vi "Magnetic Sweep 1.6.vi"() -> ()   [LabVIEW 2011]
uses:
  <vilib>/Math Plots/3D Math Plots/3D Scatter/3D Scatter XCtrl/3D Scatter.xctl
  <vilib>/Math Plots/3D Math Plots/3D Scatter/3D Scatter Datatype/Public/Plot Helper (Vector).vi
  <vilib>/Math Plots/3D Math Plots/3D Scatter/3D Scatter Datatype/3D Scatter Datatype.lvclass
panel:
  out "3D Scatter (ramp up)":refnum<class "3D Plot Datatype.lvclass">[](xcontrol)
  out "3D Scatter (ramp down)":refnum<class "3D Plot Datatype.lvclass">[](xcontrol)
  out "Heater":bool
  out "Persistent switch ready":bool
  out "error out 6":errorcluster
  in  "Temperature\nlower limite":dbl
  out "Ramping rate command":string
  out "Target field command":string
  out "error out 5":errorcluster
  in  "error out 4":errorcluster
  out "String":string="Persistent switch is not on"
  in  "Set parameter":bool
  out "status":string
  out "PID command":string
  out "setpoint command":string
  out "setpoint":dbl
  in  "stop":bool
  out "error out 3":errorcluster
  out "error out 2":errorcluster
  in  "Contour plot (ramp down)":path
  in  "Raw data (ramp down)":path
  out "Elapsed Time (s)":dbl
  out "Iteration":i32
  in  "error out":errorcluster
  out "Initial Temperature":string
  out "Zero field reached":bool
  out "Target field reached":bool
  in  "Temperature\nupper limite":dbl
  in  "Temperature\nramping step":dbl
  in  "Heater range":i16(ring) items=["High", "Medium", "Low"]
  in  "D gain":dbl
  in  "I gain":dbl
  in  "P gain":dbl
  in  "Contour plot (ramp up)":path
  out "Time elapsed":string
  in  "Timer":bool caption="Reset"
  in  "date format":enum16{"short", "long", "abbreviated"}(ring)
  in  "Save":bool
  in  "Raw data (ramp  up)":path
  out "Temperature vs Time":cluster{dbl[], dbl[]}(graph)
  out "current time":timestamp
  out "Magnetic\nField":cluster{dbl[], dbl[]}(graph)
  out "Current Resistance":string
  out "Current Temperature":string
  out "Current Field":string
  out "Status":string
  in  "Field Sweep":bool
  in  "Magnetic field\nRamp rate":dbl
  in  "Traget Field":dbl
  out "Init Response":string
  in  "error in (no error)":errorcluster
  in  "IP Address":string
  in  "Ramp":bool
  in  "Update":bool
  in  "Ramp to Zero":bool
  in  "P Switch":bool
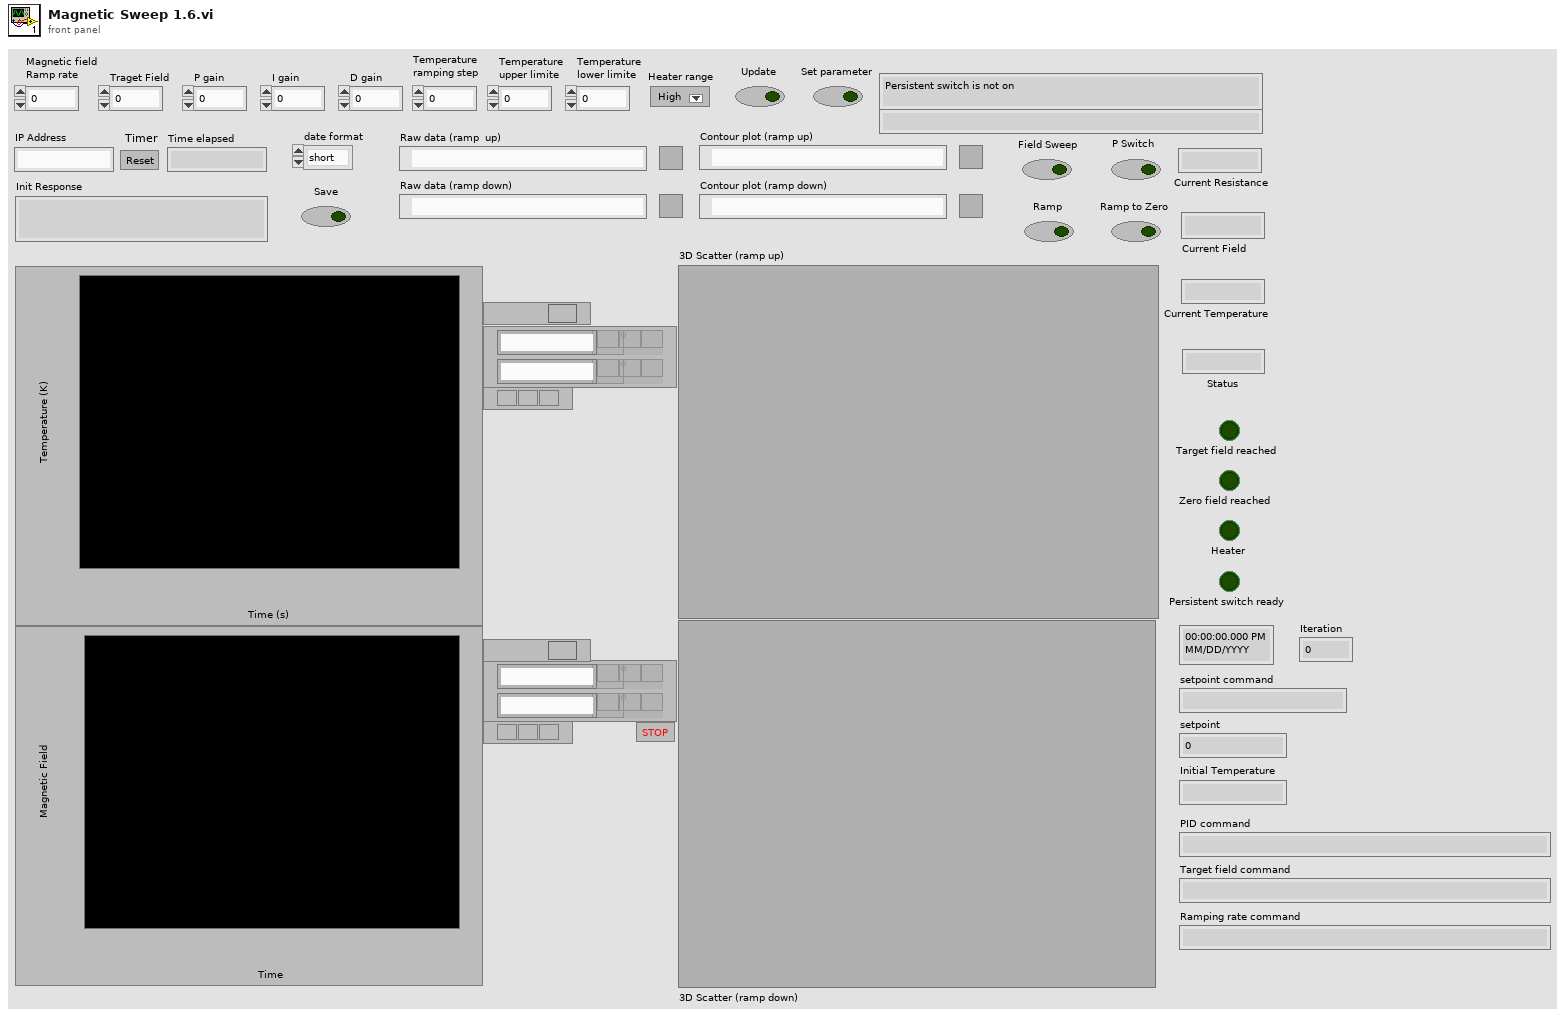
[diagram p1: front panel]
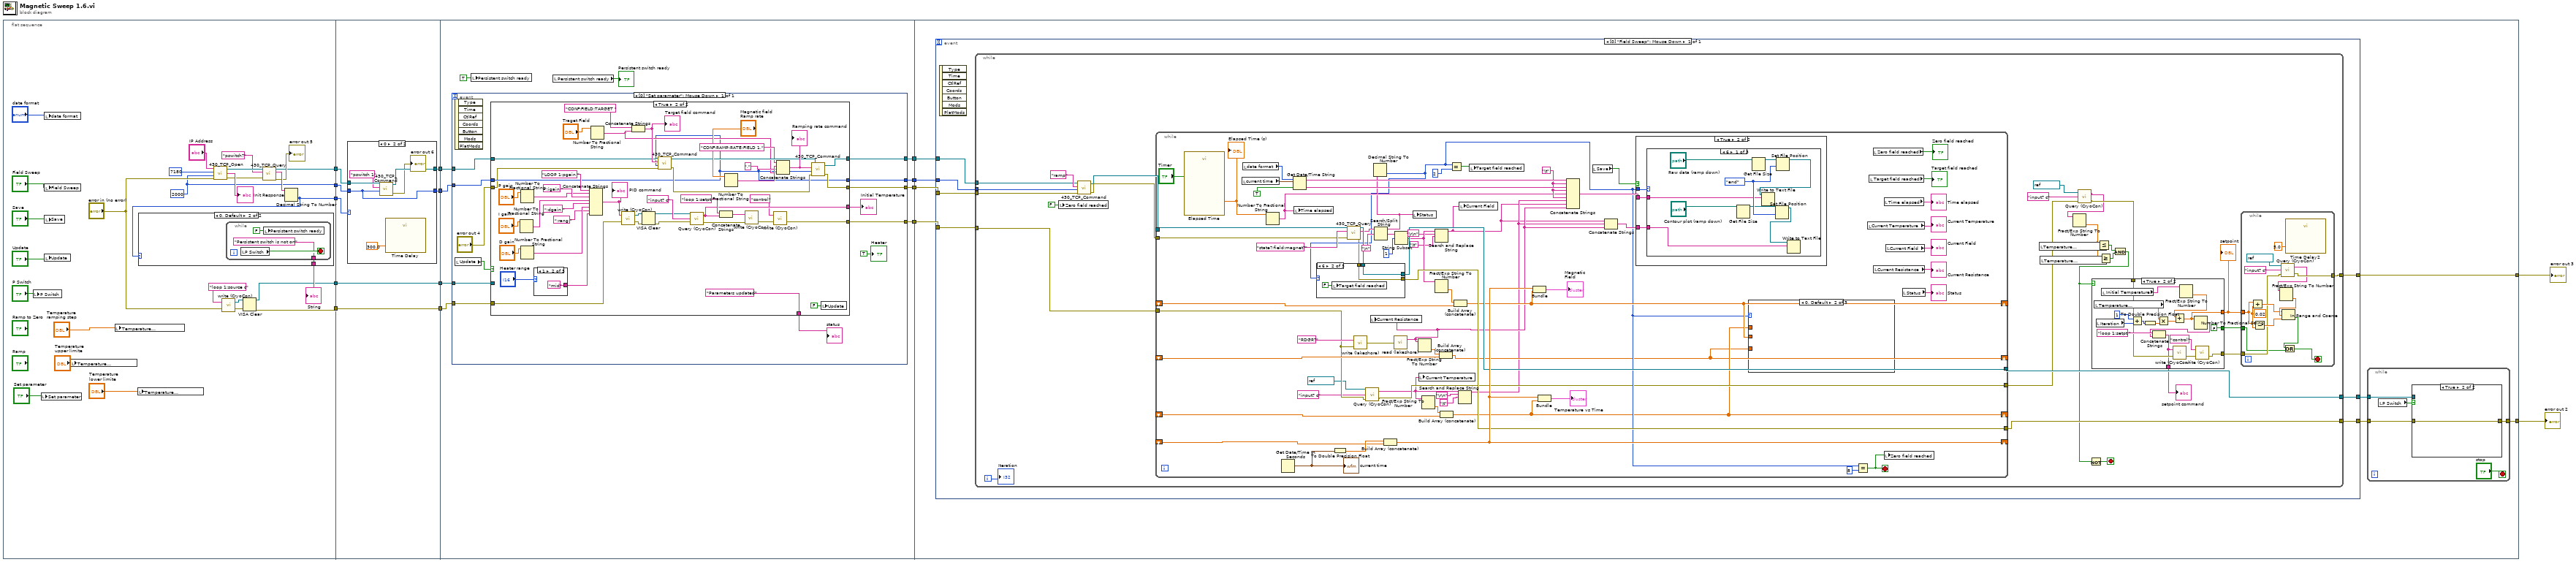
[diagram p0: block diagram]
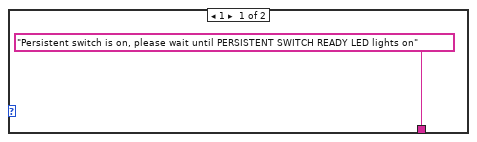
[diagram p2: hidden frame]
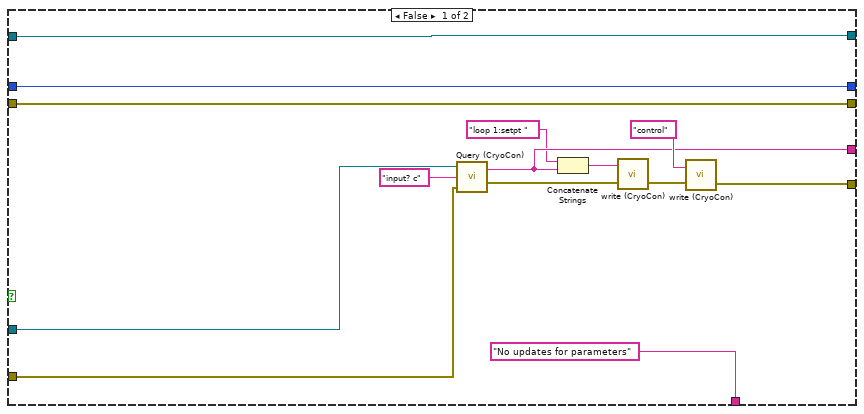
[diagram p4: hidden frame]
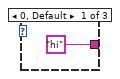
[diagram p5: hidden frame]
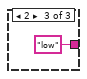
[diagram p6: hidden frame]
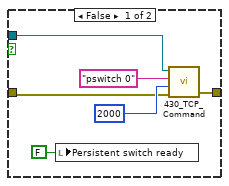
[diagram p7: hidden frame]
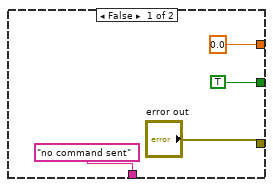
[diagram p8: hidden frame]
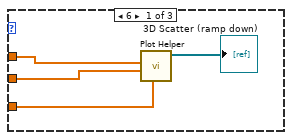
[diagram p9: hidden frame]
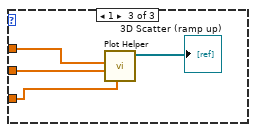
[diagram p10: hidden frame]
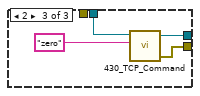
[diagram p12: hidden frame]
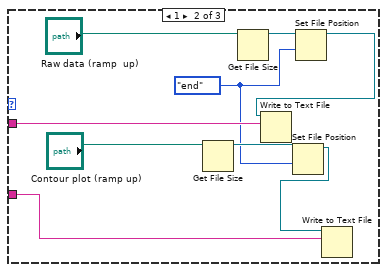
[diagram p14: hidden frame]
diagram:
  n1 = flat-sequence {
    tunnel: [w17] -> w9
    tunnel: [w20] -> w7
    tunnel: [w23] -> w5
    tunnel: [w21] -> w3
    tunnel: [w16] -> w1
    tunnel: w9 -> [w52]
    tunnel: [w50] -> w8
    tunnel: w7 -> [w51]
    tunnel: [w48] -> w6
    tunnel: w5 -> [w54]
    tunnel: [w54] -> w4
    tunnel: w3 -> [w53]
    tunnel: [w53] -> w2
    tunnel: w1 -> [w49]
    tunnel: w8 -> [w72]
    tunnel: w6 -> [w71]
    tunnel: w4 -> [w70]
    tunnel: [w69] -> w15
    tunnel: [w68] -> w12
    tunnel: [w67] -> w11
    tunnel: [w66] -> w10
    tunnel: w2 -> [w65]
    tunnel: w15 -> [w154]
    tunnel: [w153] -> w14
    tunnel: [w151] -> w13
    tunnel: w12 -> [w149]
    tunnel: w11 -> [w148]
    tunnel: w10 -> [w147]
    frame #0 {
      w20 = 2000 ("Timeout")
      n2 = local write "P Switch"("P Switch") -> ()
      n3 = local write "Set parameter"("Set parameter") -> ()
      n4 = local write "date format"("date format") -> ()
      n5 = local write "Field Sweep"("Field Sweep") -> ()
      n6 = local write "Save"("Save") -> ()
      n7 = local write "Update"("Update") -> ()
      n8 = local write "Temperature\nupper limite"("Temperature\nupper limite") -> ()
      n9 = local write "Temperature\nramping step"("Temperature\nramping step") -> ()
      n10 = local write "Temperature\nlower limite"("Temperature\nlower limite") -> ()
      n11 = call "430_TCP_Open.vi"("IP Address"="IP Address", "TCP Port"=7180, "timeout ms (2000)"=w20, "error in (no error)"="error in (no error)") -> ("connection ID"=w30:refnum<k5>, "Init Response"=→"Init Response":string, "error out"=w29:errorcluster)  [unwired: 2 in]
      n12 = call "write (CryoCon).vi"("error in (no error)"="error in (no error)", "write buffer"="loop 1:source c") -> ("error out"=w25:errorcluster, "VISA resource name out"=w24:refnum<visa-resource-name>)
      n13 = VISA Clear(VISA resource name=w24, error in (no error)=w25) -> (VISA resource name out=w21:refnum<visa-resource-name>, error out=w23:errorcluster)
      n14 = call "430_TCP_Query.vi"("error in (no error)"=w29, "Command"="pswitch?", "connection ID"=w30) -> ("error out"=→"error out 5":errorcluster, "Response"=w27:string, "connection ID out"=w17:refnum<k5>)  [unwired: 4 in, 2 out]
      n15 = Decimal String To Number(string=w27) -> (number=w16:i32)  [unwired: 2 in, 1 out]
      n16 = case shown="0, Default" w16 {
        tunnel: ["Persistent switch is on, please wait until PERSISTENT SWITCH READY LED lights on" w44] -> w22
        frame 1 {
        }
        frame 0, Default {
          n17 = while {
            tunnel: ["Persistent switch is not on"] -> w44
            stop <- w47 stop-if-true
            n18 = local read "P Switch"() -> (w47:bool)
            n19 = local write "Persistent switch ready"(FALSE ("Persistent switch ready")) -> ()
          }
        }
      }
      "String" <- w22
    }
    frame #1 {
      n20 = case shown="0" w49 {
        tunnel: w52 -> [w56 w62]
        tunnel: w51 -> [w55 w57]
        tunnel: [w56 w61] -> w50
        tunnel: [w55 w57] -> w48
        frame 1, Default {
        }
        frame 0 {
          n21 = call "430_TCP_Command.vi"("Timeout"=w57, "Command"="pswitch 1", "connection ID"=w62) -> ("error out"=→"error out 6":errorcluster, "connection ID out"=w61:refnum<k5>)  [unwired: 1 in, 1 out]
          n22 = call "Time Delay"("Delay Time (s)"=300.0) -> ()  [unwired: 10 in, 1 out]
        }
      }
    }
    frame #2 {
      n23 = event shown="[0] \"Set parameter\": Mouse Down" {
        selector: _ -> [_]
        dyn-events: _ -> [_]
        timeout: _ -> [_]
        tunnel: w72 -> [w85]
        tunnel: w71 -> [w84]
        tunnel: w70 -> [w83]
        tunnel: [w82] -> w69
        tunnel: [w81] -> w68
        tunnel: [w80] -> w67
        tunnel: [w79] -> w66
        tunnel: w65 -> [w75]
        event "Set parameter": Mouse Down {
          n24 = event-data() -> ()  [unwired: 1 in, 7 out]
          n25 = local read "Update"() -> (w76:bool)
          n26 = case shown="True" w76 {
            tunnel: w85 -> [w97 w141]
            tunnel: w84 -> [w98 w113]
            tunnel: w83 -> [w94 w120]
            tunnel: [w86 w101] -> w82
            tunnel: ["No updates for parameters" ("String") "Parameters updated" ("String")] -> w78
            tunnel: [w93 w115] -> w81
            tunnel: [w97 w114] -> w80
            tunnel: [w98 w113] -> w79
            tunnel: [w89 w105] -> w77
            tunnel: w75 -> [w95 _]
            tunnel: "error out 4" -> [w93 w100]
            frame False {
              n27 = call "Query (CryoCon).vi"("error in (no error)"=w94, "write buffer"="input? c", "VISA resource name 2"=w95) -> ("error out"=w87:errorcluster, "read buffer"=w89:string)
              n28 = Concatenate Strings("loop 1:setpt " ("write buffer"), w89) -> (w92:string)
              n29 = call "write (CryoCon).vi"("error in (no error)"=w87, "write buffer"=w92) -> ("error out"=w91:errorcluster)  [unwired: 1 out]
              n30 = call "write (CryoCon).vi"("error in (no error)"=w91, "write buffer"="control") -> ("error out"=w86:errorcluster)  [unwired: 1 out]
            }
            frame True {
              n31 = Number To Fractional String(number="I gain") -> (F-format string=w124:string)  [unwired: 3 in]
              n32 = Number To Fractional String(number="D gain") -> (F-format string=w122:string)  [unwired: 3 in]
              n33 = Number To Fractional String(number="P gain") -> (F-format string=w125:string)  [unwired: 3 in]
              n34 = case shown="1" "Heater range" {
                tunnel: ["hi" "mid" "low"] -> w117
                frame 0, Default {
                }
                frame 1 {
                }
                frame 2 {
                }
              }
              n35 = Concatenate Strings("LOOP 1:pgain " ("write buffer"), w125, ";igain " ("string"), w124, ";dgain " ("string"), w122, ";rang " ("string"), w117) -> (w121:string)
              "PID command" <- w121
              n36 = Number To Fractional String(number="Traget Field") -> (F-format string=w131:string)  [unwired: 3 in]
              n37 = call "write (CryoCon).vi"("error in (no error)"=w120, "write buffer"=w121) -> ("error out"=w112:errorcluster, "VISA resource name out"=w111:refnum<visa-resource-name>)
              n38 = Concatenate Strings("CONF:FIELD:TARGET ", w131) -> (w142:string)
              "Target field command" <- w142
              n39 = VISA Clear(VISA resource name=w111, error in (no error)=w112) -> (VISA resource name out=w108:refnum<visa-resource-name>, error out=w109:errorcluster)
              n40 = call "430_TCP_Command.vi"("error in (no error)"=w100, "Timeout"=w113, "Command"=w142, "connection ID"=w141) -> ("error out"=w140:errorcluster, "connection ID out"=w136:refnum<k5>)  [unwired: 1 out]
              n41 = call "Query (CryoCon).vi"("error in (no error)"=w109, "write buffer"="input? c", "VISA resource name 2"=w108) -> ("error out"=w107:errorcluster, "read buffer"=w105:string)
              n42 = Concatenate Strings("loop 1:setpt " ("write buffer"), w105) -> (w104:string)
              n43 = Number To Fractional String(number="Magnetic field\nRamp rate") -> (F-format string=w134:string)  [unwired: 3 in]
              n44 = call "write (CryoCon).vi"("error in (no error)"=w107, "write buffer"=w104) -> ("error out"=w103:errorcluster)  [unwired: 1 out]
              n45 = call "write (CryoCon).vi"("error in (no error)"=w103, "write buffer"="control") -> ("error out"=w101:errorcluster)  [unwired: 1 out]
              n46 = Concatenate Strings("CONF:RAMP:RATE:FIELD 1," ("string"), w134, "," ("string"), w131) -> (w137:string)
              "Ramping rate command" <- w137
              n47 = call "430_TCP_Command.vi"("error in (no error)"=w140, "Timeout"=w113, "Command"=w137, "connection ID"=w136) -> ("error out"=w115:errorcluster, "connection ID out"=w114:refnum<k5>)  [unwired: 1 out]
              n48 = local write "Update"(FALSE ("Update")) -> ()
            }
          }
          "Initial Temperature" <- w77
          "status" <- w78
          "Heater" <- TRUE ("Heater")
        }
      }
      n49 = local write "Persistent switch ready"(TRUE ("Persistent switch ready")) -> ()
      n50 = local read "Persistent switch ready"() -> (→"Persistent switch ready":bool)
    }
    frame #3 {
      n51 = event shown="[0] \"Field Sweep\": Mouse Down" {
        selector: _ -> [_]
        dyn-events: _ -> [_]
        timeout: _ -> [_]
        tunnel: w154 -> [w173]
        tunnel: [w172] -> w153
        tunnel: [w171] -> w152
        tunnel: [w170] -> w150
        tunnel: w149 -> [w169]
        tunnel: w148 -> [w168]
        tunnel: w147 -> [w167]
        event "Field Sweep": Mouse Down {
          n52 = event-data() -> ()  [unwired: 1 in, 7 out]
          n53 = while {
            tunnel: w173 -> [w199]
            tunnel: [w191] -> w172
            tunnel: [w190] -> w171
            tunnel: [w189] -> w170
            tunnel: w169 -> [w187]
            tunnel: w168 -> [w186]
            tunnel: w167 -> [w185]
            i -> [w196]
            stop <- w192 stop-if-true
            n54 = local write "Zero field reached"(FALSE ("Zero field reached")) -> ()
            n55 = call "430_TCP_Command.vi"("error in (no error)"=w187, "Timeout"=w185, "Command"="ramp", "connection ID"=w186) -> ("error out"=w201:errorcluster, "connection ID out"=w200:refnum<k5>)  [unwired: 1 out]
            n56 = while {
              shift-right: [w256] -> _
              shift-left: _ -> [w296]
              shift-right: [w243] -> _
              shift-left: _ -> [w301]
              shift-right: [w242] -> _
              shift-left: _ -> [w298]
              shift-right: [w293] -> _
              shift-left: _ -> [w239]
              tunnel: w201 -> [w283]
              tunnel: w200 -> [w282]
              tunnel: w199 -> [w253]
              tunnel: [w252] -> w183
              tunnel: [w264] -> w190
              tunnel: [w263] -> w189
              stop <- w266 stop-if-true
              w287 = "\t"
              n57 = call "Elapsed Time"("Reset"="Timer") -> ("Elapsed Time (s)"=w277:dbl)  [unwired: 11 in, 7 out]
              "Elapsed Time (s)" <- w277
              n58 = local read "current time"() -> (w285:timestamp)
              n59 = local read "date format"() -> (w279:enum16{"short", "long", "abbreviated"})
              n60 = Number To Fractional String(number=w277) -> (F-format string=w280:string)  [unwired: 3 in]
              n61 = Get Date/Time In Seconds() -> (seconds since 1Jan1904=w276:timestamp)
              "current time" <- w276
              n62 = Get Date/Time String(date format (0)=w279, seconds (now)=w285, want seconds? (F)=TRUE) -> (date string=w289:string, time string=w288:string)
              n63 = local write "Time elapsed"(w280) -> ()
              n64 = To Double Precision Float(number=w276) -> (double precision float=w240:dbl)
              n65 = call "430_TCP_Query.vi"("error in (no error)"=w283, "Command"="state?;field:magnet?", "connection ID"=w282) -> ("error out"=w254:errorcluster, "Response"=w262:string, "connection ID out"=w265:refnum<k5>)  [unwired: 4 in, 2 out]
              n66 = call "write (lakeshore).vi"("error in (no error)"=w253, "write buffer"="RDGR?") -> ("error out"=w300:errorcluster)
              n67 = call "Query (CryoCon).vi"("error in (no error)"=w253, "write buffer"="input? c", "VISA resource name 2"=refnum<visa-resource-name> "COM3") -> ("error out"=w252:errorcluster, "read buffer"=w249:string)
              n68 = Search/Split String(string=w262, search string/char (-)="\n") -> (substring before match=w261:string, match + rest of string=w260:string)  [unwired: 1 in, 1 out]
              n69 = Decimal String To Number(string=w261) -> (number=w255:i32)  [unwired: 2 in, 1 out]
              n70 = case shown="6" w255 {
                tunnel: [w311 w313 w318] -> w263
                tunnel: w265 -> [w312 w315 w317]
                tunnel: [w312 w315 w316] -> w264
                tunnel: w254 -> [w311 w313 _]
                frame 0, Default {
                }
                frame 6 {
                  n71 = local write "Target field reached"(FALSE ("Target field reached")) -> ()
                }
                frame 2 {
                  n72 = call "430_TCP_Command.vi"("Command"="zero", "connection ID"=w317) -> ("error out"=w318:errorcluster, "connection ID out"=w316:refnum<k5>)  [unwired: 2 in, 1 out]
                }
              }
              n73 = Build Array (concatenate)(w240, w239) -> (w293:dbl[])
              n74 = call "read (lakeshore).vi"("error in (no error)"=w300) -> ("read buffer"=w241:string)  [unwired: 1 out]
              n75 = local write "Current Resistance"(w241) -> ()
              n76 = String Subset(string=w260, offset (0)=1) -> (substring=w246:string)  [unwired: 1 in]
              n77 = local write "Status"(w261) -> ()
              n78 = Fract/Exp String To Number(string=w241) -> (number=w294:dbl)  [unwired: 3 in, 1 out]
              n79 = local write "Current Temperature"(w249) -> ()
              n80 = Fract/Exp String To Number(string=w249) -> (number=w295:dbl)  [unwired: 3 in, 1 out]
              n81 = Search and Replace String(input string=w246, search string="\r\n", replace string="\t") -> (result string=w237:string)  [unwired: 5 in, 3 out]
              n82 = Fract/Exp String To Number(string=w246) -> (number=w297:dbl)  [unwired: 3 in, 1 out]
              n83 = Build Array (concatenate)(w294, w298) -> (w242:dbl[])
              n84 = Build Array (concatenate)(w295, w301) -> (w243:dbl[])
              n85 = Equal?(x=w255, y=2) -> (x = y?=w281:bool)
              n86 = Build Array (concatenate)(w297, w296) -> (w256:dbl[])
              n87 = Search and Replace String(input string=w249, search string="\r\n", replace string="\t") -> (result string=w238:string)  [unwired: 5 in, 3 out]
              n88 = local write "Current Field"(w237) -> ()
              n89 = local write "Target field reached"(w281) -> ()
              n90 = Bundle(w293, w256) -> (→"Magnetic\nField":cluster{dbl[], dbl[]})  [unwired: 1 in]
              n91 = Bundle(w293, w243) -> (→"Temperature vs Time":cluster{dbl[], dbl[]})  [unwired: 1 in]
              n92 = Concatenate Strings(w289, w287, w288, w287, w280, w287, w238, w237, w241) -> (w292:string)
              n93 = local read "Save"() -> (w275:bool)
              n94 = Concatenate Strings(w237, w238, w241) -> (w286:string)
              n95 = case shown="True" w275 {
                tunnel: w292 -> [_ w322]
                tunnel: w286 -> [_ w321]
                tunnel: w255 -> [_ w320]
                frame False {
                }
                frame True {
                  n96 = case shown="6" w320 {
                    tunnel: w322 -> [w324 w340 _]
                    tunnel: w321 -> [w323 w334 _]
                    frame 6 {
                      w330 = enum16{"start", "end", "current"}."end" ("from (0:start)")
                      n97 = Get File Size(file="Contour plot (ramp down)") -> (refnum out=w329:refnum<file>)  [unwired: 1 in, 2 out]
                      n98 = Get File Size(file="Raw data (ramp down)") -> (refnum out=w326:refnum<file>)  [unwired: 1 in, 2 out]
                      n99 = Set File Position(refnum=w329, from (0:start)=w330) -> (refnum out=w331:refnum<file>)  [unwired: 2 in, 1 out]
                      n100 = Set File Position(refnum=w326, from (0:start)=w330) -> (refnum out=w327:refnum<file>)  [unwired: 2 in, 1 out]
                      n101 = Write to Text File(file (use dialog)=w327, text=w324) -> ()  [unwired: 2 in, 3 out]
                      n102 = Write to Text File(file (use dialog)=w331, text=w323) -> ()  [unwired: 2 in, 3 out]
                    }
                    frame 1 {
                      w333 = enum16{"start", "end", "current"}."end" ("from (0:start)")
                      n103 = Get File Size(file="Contour plot (ramp up)") -> (refnum out=w335:refnum<file>)  [unwired: 1 in, 2 out]
                      n104 = Get File Size(file="Raw data (ramp  up)") -> (refnum out=w338:refnum<file>)  [unwired: 1 in, 2 out]
                      n105 = Set File Position(refnum=w335, from (0:start)=w333) -> (refnum out=w332:refnum<file>)  [unwired: 2 in, 1 out]
                      n106 = Set File Position(refnum=w338, from (0:start)=w333) -> (refnum out=w337:refnum<file>)  [unwired: 2 in, 1 out]
                      n107 = Write to Text File(file (use dialog)=w337, text=w340) -> ()  [unwired: 2 in, 3 out]
                      n108 = Write to Text File(file (use dialog)=w332, text=w334) -> ()  [unwired: 2 in, 3 out]
                    }
                    frame Default {
                    }
                  }
                }
              }
              n109 = case shown="0, Default" w255 {
                tunnel: w243 -> [w304 _ w307]
                tunnel: w256 -> [w303 _ w308]
                tunnel: w242 -> [w305 _ w309]
                frame 6 {
                  n110 = call-poly <vilib>:"Plot Helper.vi"("z vector"=w305, "y vector"=w303, "x vector"=w304) -> ("3D Plot lvclass Array out"=→"3D Scatter (ramp down)":refnum<class "3D Plot Datatype.lvclass">[])  [unwired: 3 in, 5 out]
                }
                frame 0, Default {
                }
                frame 1 {
                  n111 = call-poly <vilib>:"Plot Helper.vi"("z vector"=w309, "y vector"=w308, "x vector"=w307) -> ("3D Plot lvclass Array out"=→"3D Scatter (ramp up)":refnum<class "3D Plot Datatype.lvclass">[])  [unwired: 3 in, 5 out]
                }
              }
              n112 = Equal?(x=w255, y=8) -> (x = y?=w266:bool)
              n113 = local read "Current Temperature"() -> (→"Current Temperature":string)
              n114 = local read "Target field reached"() -> (→"Target field reached":bool)
              n115 = local read "Zero field reached"() -> (→"Zero field reached":bool)
              n116 = local read "Current Resistance"() -> (→"Current Resistance":string)
              n117 = local read "Time elapsed"() -> (→"Time elapsed":string)
              n118 = local write "Zero field reached"(w266) -> ()
              n119 = local read "Current Field"() -> (→"Current Field":string)
              n120 = local read "Status"() -> (→"Status":string)
            }
            n121 = local read "Temperature\nupper limite"() -> (w193:dbl)
            n122 = local read "Temperature\nlower limite"() -> (w178:dbl)
            n123 = call "Query (CryoCon).vi"("error in (no error)"=w183, "write buffer"="input? c", "VISA resource name 2"=refnum<visa-resource-name> "COM3") -> ("error out"=w182:errorcluster, "read buffer"=w181:string)
            n124 = Fract/Exp String To Number(string=w181) -> (number=w179:dbl)  [unwired: 3 in, 1 out]
            n125 = Less Or Equal?(x=w179, y=w193) -> (x <= y?=w176:bool)
            n126 = Greater Or Equal?(x=w179, y=w178) -> (x >= y?=w177:bool)
            n127 = And(x=w176, y=w177) -> (x .and. y?=w175:bool)
            n128 = Not(x=w175) -> (.not. x?=w192:bool)
            n129 = case shown="True" w175 {
              tunnel: w182 -> [_ w234]
              tunnel: ["error out" w223] -> w198
              tunnel: [0.0 w231] -> w197
              tunnel: ["no command sent" w227] -> w188
              tunnel: [TRUE FALSE] -> w174
              frame False {
              }
              frame True {
                n130 = local read "Temperature\nramping step"() -> (w229:dbl)
                n131 = local read "Iteration"() -> (w226:i32)
                n132 = local read "Initial Temperature"() -> (w233:string)
                n133 = Add(x=1, y=w226) -> (x+y=w225:i32)
                n134 = To Double Precision Float(number=w225) -> (double precision float=w228:dbl)
                n135 = Multiply(x=w229, y=w228) -> (x*y=w230:dbl)
                n136 = Fract/Exp String To Number(string=w233) -> (number=w232:dbl)  [unwired: 3 in, 1 out]
                n137 = Add(x=w232, y=w230) -> (x+y=w231:dbl)
                n138 = Number To Fractional String(number=w231) -> (F-format string=w235:string)  [unwired: 3 in]
                n139 = Concatenate Strings("loop 1:setpt " ("write buffer"), w235) -> (w227:string)
                n140 = call "write (CryoCon).vi"("error in (no error)"=w234, "write buffer"=w227) -> ("error out"=w222:errorcluster)  [unwired: 1 out]
                n141 = call "write (CryoCon).vi"("error in (no error)"=w222, "write buffer"="control") -> ("error out"=w223:errorcluster)  [unwired: 1 out]
              }
            }
            "setpoint" <- w197
            "setpoint command" <- w188
            n142 = while {
              tunnel: w198 -> [w208]
              tunnel: w197 -> [w214]
              tunnel: [w207] -> w191
              tunnel: w174 -> [w204]
              stop <- w202 stop-if-true
              w211 = 0.02 ("y")
              n143 = Add(x=w214, y=w211) -> (x+y=w213:dbl)
              n144 = Subtract(x=w214, y=w211) -> (x-y=w212:dbl)
              n145 = call "Query (CryoCon).vi"("error in (no error)"=w208, "write buffer"="input? c", "VISA resource name 2"=refnum<visa-resource-name> "COM3") -> ("error out"=w207:errorcluster, "read buffer"=w206:string)
              n146 = Fract/Exp String To Number(string=w206) -> (number=w215:dbl)  [unwired: 3 in, 1 out]
              n147 = In Range and Coerce(upper limit=w213, x=w215, lower limit=w212) -> (In Range?=w203:bool)  [unwired: 1 out]
              n148 = Or(x=w203, y=w204) -> (x .or. y?=w202:bool)
              n149 = call "Time Delay2"("Delay Time (s)"=5.0) -> ()  [unwired: 10 in, 1 out]
            }
            "Iteration" <- w196
          }
        }
      }
      n150 = while {
        tunnel: w152 -> [w159]
        tunnel: [w157] -> w151
        tunnel: w150 -> [w156]
        stop <- "stop" stop-if-true
        n151 = local read "P Switch"() -> (w158:bool)
        n152 = case shown="True" w158 {
          tunnel: w159 -> [w164 _]
          tunnel: [w162 w166] -> w157
          tunnel: w156 -> [w161 w166]
          frame False {
            n153 = local write "Persistent switch ready"(FALSE ("Persistent switch ready")) -> ()
            n154 = call "430_TCP_Command.vi"("error in (no error)"=w161, "Timeout"=2000, "Command"="pswitch 0", "connection ID"=w164) -> ("error out"=w162:errorcluster)  [unwired: 2 out]
          }
          frame True {
          }
        }
      }
    }
  }
  "error out 2" <- w13
  "error out 3" <- w14
